vi "CIC_downsample4.vi"(8 "valid in":bool, 10 "din":fxp<+/-,20,16>) -> (0 "valid out":bool, 1 "rdy for data":bool, 2 "dout":fxp<+/-,25,19>)   [LabVIEW 2013]
uses:
  <vilib>/rvi/FXPMathLib/FxpConvert/subVIs/nifxpmath_Convert_SimConfig.ctl
  <vilib>/fxp/LVFixedPointQuantizationPolicyTypeDef.ctl
  <vilib>/fxp/LVFixedPointOverflowPolicyTypeDef.ctl
  <vilib>/rvi/FXPMathLib/FxpConvert/simVIs/DllFxpConvertTemp_sub.vi
  <vilib>/rvi/IPIntegrationNode/IPINode_Utilities/niFpgaIPINodeSimCore.vi
  <vilib>/rvi/FXPMathLib/FxpConvert/XNode/nifxpmath_Convert.xnode
  <vilib>/rvi/XilinxIP/XIPIN_XNode/niFpgaXIPIN.xnode
  CIC_downsample4/CIC Downsample4/CIC_Downsample4_E9B3D0256E9345788E26D47FE8F7B586.dll
  <vilib>/rvi/IPIntegrationNode/IPINode_Xnode/niFpgaIPINode.xnode
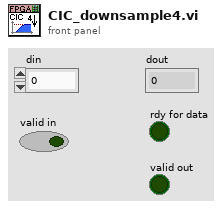
[diagram p1: front panel]
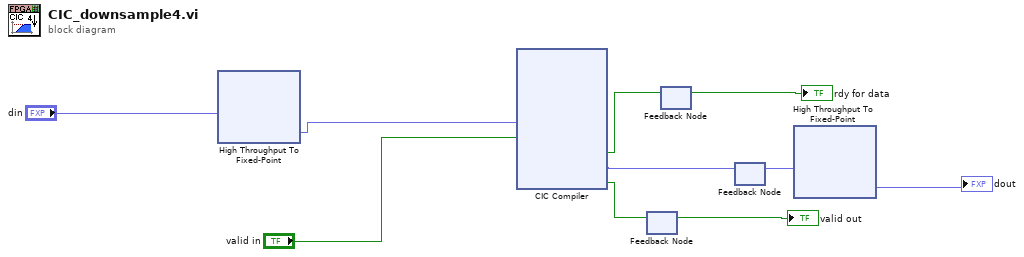
[diagram p0: block diagram]
diagram:
  n1 = xnode "High Throughput To Fixed-Point"("x"="din") -> ("y"=w8:fxp<+/-,24,20>)
  n2 = xnode ("CIC Compiler")("s_axis_data_tdata"=w8, "s_axis_data_tvalid"="valid in") -> ("s_axis_data_tready"=w1:bool, "m_axis_data_tdata"=w6:fxp<+/-,32,18>, "m_axis_data_tvalid"=w4:bool)  [unwired: 2 in]
  n3 = feedback #1() -> (→"valid out":bool)  [unwired: 1 in]
  n4 = feedback-in #1(w4) -> ()
  n5 = feedback #2() -> (→"rdy for data":bool)  [unwired: 1 in]
  n6 = feedback-in #2(w1) -> ()
  n7 = feedback #3() -> (w7:fxp<+/-,32,18>)  [unwired: 1 in]
  n8 = feedback-in #3(w6) -> ()
  n9 = xnode "High Throughput To Fixed-Point"("x"=w7) -> ("y"=→"dout":fxp<+/-,25,19>)
